vi "Proyecto 1 Control de Entrada.vi"() -> ()   [LabVIEW 2015]
panel:
  in  "Tab Control":T1(tab)
  in  "stop":bool
  out "Entradas/Salidas":i64
  out "Entrada":bool=TRUE
  out "Salida":bool=TRUE
  in  "Ajuste de Apertura":i32(knob)=3 scale=0.0..10.0
  in  "Control de Velocidad":i16(knob)=5 scale=0.0..10.0
  in  "Tiempo de espera":i16(knob)=1 scale=0.0..10.0
  # "Control Automatizado de Entrada"
  # "Componentes utilizados:\n      -Resistencias: 330 Ohms x2, 2.2 KOhms x2 a 1/2 watt\n      -Sensor infrarrojo y receptor infrarrojo\n      -LM293D(Puente H)\n      -Motor a pasos: M42SP-6TG (12 volts)\n      -Fuente de alimentación dual de 5 y 12 Volts"
  # "Serrano Bermúdez Luis Esteban"
  # "4/5/2019"
  # "Control de Entradas/Salidas a travez\nde sensores infrarrojos de obstrucción\ny de un motor a pasos que es controlado\na partir de un módulo LM293D (Conocido\ncomunmente como puente H)"
  # "Tiempo de Espera: Controla el tiempo que \npermanecerá abierta la puerta.\nControl de Velocidad: Ajusta la velocidad\ncon la que se mueve el motor a pasos.\nAjuste de Apertura: Modifica el grado de\napertura de la puerta permitiendo poder\naplicarlo a diferentes tipos de puertas"
  # "Entrada: Luz indicadora si se puede avanzar\na entrar o salir.\nSalida: Luz indicadora si se puede avanzar\na entrar o salir."
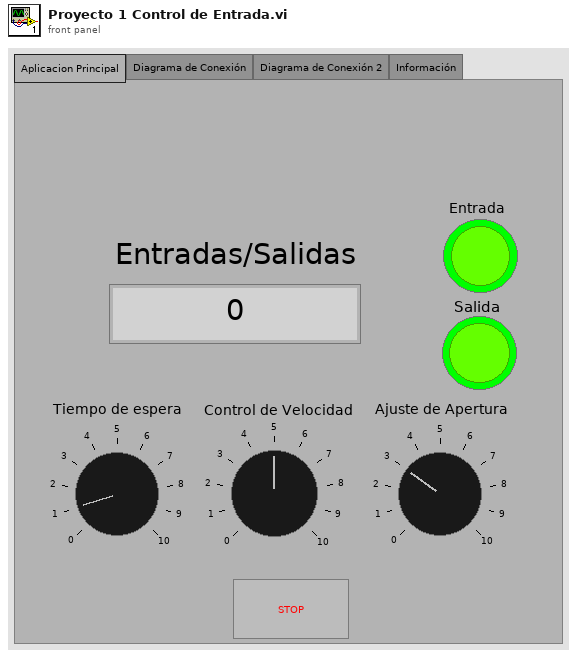
[diagram p1: front panel]
types:
  T1 = enum32{"Aplicacion Principal", "Diagrama de Conexión", "Diagrama de Conexión 2", "Información"}
  T2 = enum16{"Estado 0", "Estado 1", "Estado 2", "Estado 3"}
  T3 = enum16{"Estado 0", "Estado 1", "Estado 2", "Estado 3", "Estado 4", "Estado 5"}
  T4 = enum16{"Estado 0", "Estado 1", "Estado 2", "Estado 3", "Estado 4", "Estado 5", "Estado 6", "Estado 7", "Estado 8", "Estado 9"}
  T5 = enum16{"Estado 0", "Estado 1", "Estado 2", "Estado 3", "Estado 4", "Estado 5"}[]
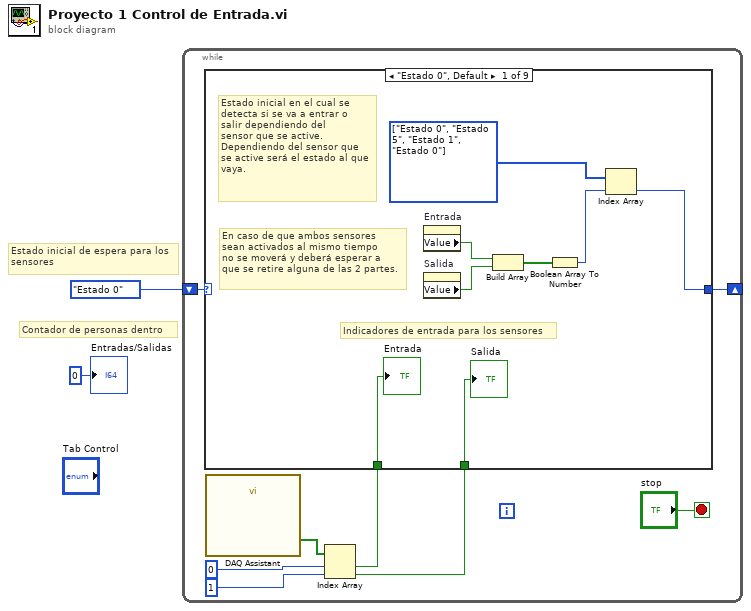
[diagram p0: block diagram]
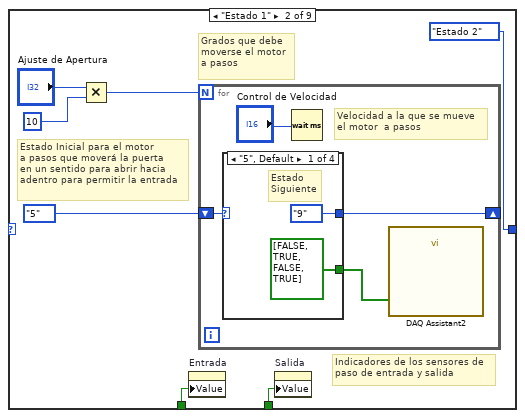
[diagram p2: hidden frame]
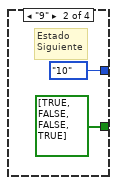
[diagram p3: hidden frame]
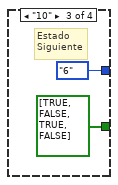
[diagram p4: hidden frame]
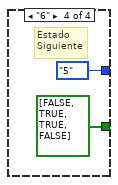
[diagram p5: hidden frame]
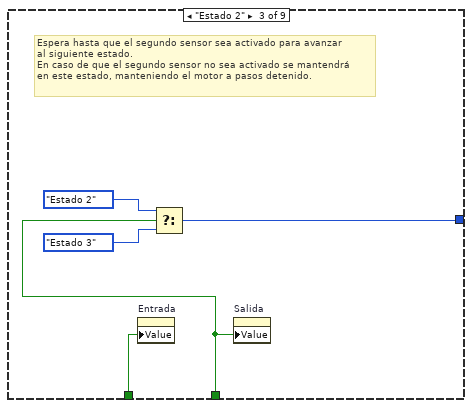
[diagram p6: hidden frame]
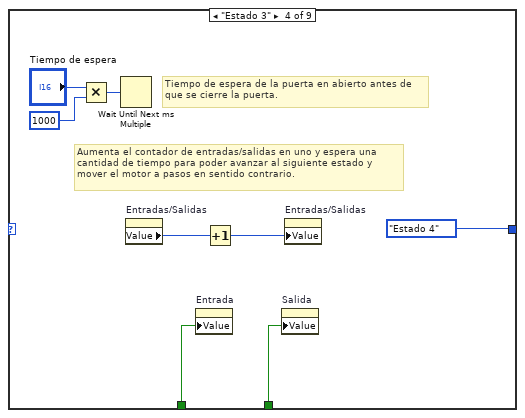
[diagram p7: hidden frame]
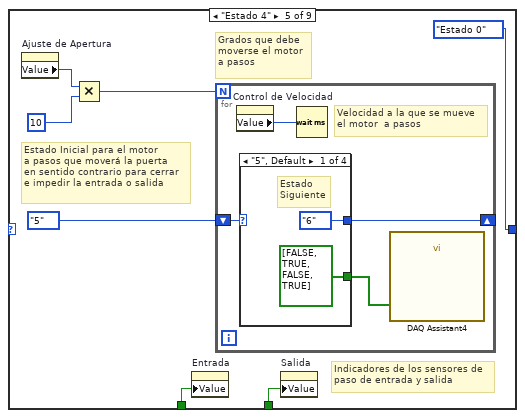
[diagram p8: hidden frame]
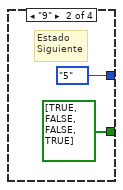
[diagram p9: hidden frame]
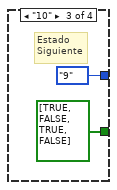
[diagram p10: hidden frame]
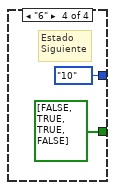
[diagram p11: hidden frame]
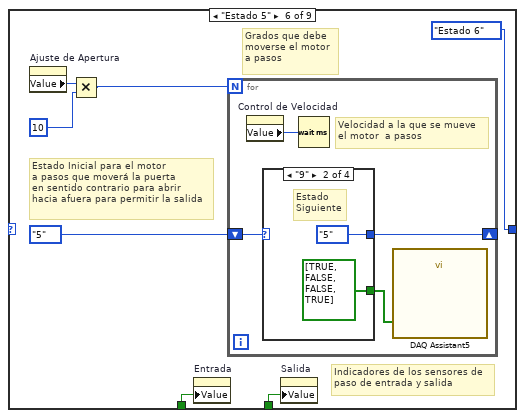
[diagram p12: hidden frame]
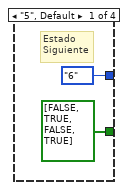
[diagram p13: hidden frame]
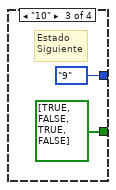
[diagram p14: hidden frame]
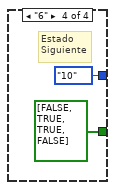
[diagram p15: hidden frame]
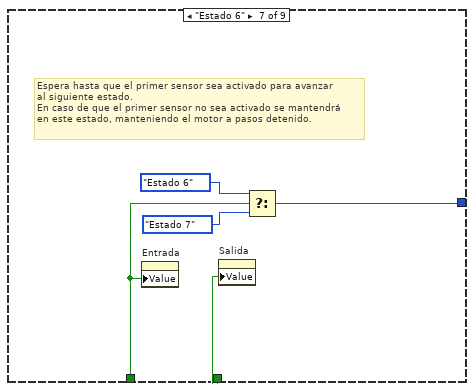
[diagram p16: hidden frame]
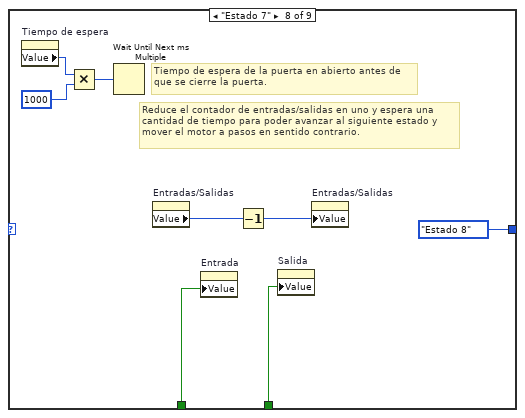
[diagram p17: hidden frame]
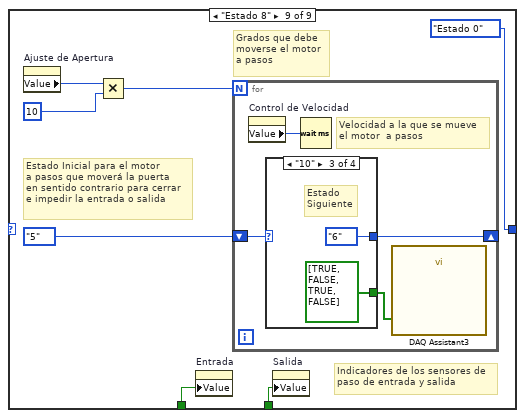
[diagram p18: hidden frame]
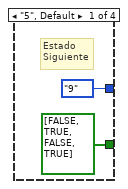
[diagram p19: hidden frame]
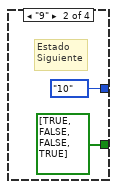
[diagram p20: hidden frame]
diagram:
  # "Contador de personas dentro"
  # "Estado inicial de espera para los\nsensores"
  n1 = while {
    shift-right: [w9] -> _
    shift-left: T2."Estado 0" -> [w10]
    stop <- "stop" stop-if-true
    n2 = call "DAQ Assistant"() -> ("data"=w5:bool[])  [unwired: 17 in, 2 out]
    n3 = Index Array(array=w5, index #1=0 ("index"), index #2=1 ("index")) -> (element #1=w4:bool, element #2=w3:bool)
    n4 = case shown="\"Estado 0\", Default" w10 {
      tunnel: [w18 T2."Estado 2" w40 T3."Estado 4" T4."Estado 0" T4."Estado 6" w91 T4."Estado 8" T4."Estado 0"] -> w9
      tunnel: w4 -> [w17 w19 w38 w46 w52 w70 w90 w97 w102]
      tunnel: w3 -> [w16 w20 w39 w47 w51 w71 w89 w98 w103]
      frame "Estado 0", Default {
        w15 = T5 [enum."Estado 0", enum."Estado 5", enum."Estado 1", enum."Estado 0"] items=["Estado 0", "Estado 1", "Estado 2", "Estado 3", "Estado 4", "Estado 5"]
        # "Indicadores de entrada para los sensores"
        # "En caso de que ambos sensores\nsean activados al mismo tiempo\nno se moverá y deberá esperar a\nque se retire alguna de las 2 partes."
        # "Estado inicial en el cual se\ndetecta si se va a entrar o\nsalir dependiendo del \nsensor que se active.\nDependiendo del sensor que\nse active será el estado al que\nvaya."
        n5 = property on="Entrada" class="Bool (strict)"() -> ("Value"=w12:bool)  [unwired: 2 in, 2 out]
        n6 = property on="Salida" class="Bool (strict)"() -> ("Value"=w11:bool)  [unwired: 2 in, 2 out]
        n7 = Build Array(w12, w11) -> (w13:bool[])
        n8 = Boolean Array To Number(Boolean array=w13) -> (number=w14:u32)
        n9 = Index Array(array=w15, index=w14) -> (element=w18:T3)
        "Entrada" <- w17
        "Salida" <- w16
      }
      frame "Estado 1" {
        # "Indicadores de los sensores de\npaso de entrada y salida"
        # "Grados que debe moverse el motor a pasos"
        # "Estado Inicial para el motor \na pasos que moverá la puerta\nen un sentido para abrir hacia\nadentro para permitir la entrada"
        n10 = Multiply(x="Ajuste de Apertura", y=10) -> (x*y=w23:i32)
        n11 = property on="Entrada" class="Bool (strict)"("Value"=w19) -> ()  [unwired: 2 in, 2 out]
        n12 = for {
          N: w23 -> [_]
          shift-right: [w28] -> _
          shift-left: enum16{"5", "9", "10", "6"}."5" -> [w29]
          # "Velocidad a la que se mueve\nel motor  a pasos"
          n13 = case shown="\"5\", Default" w29 {
            tunnel: [bool[] [FALSE, TRUE, FALSE, TRUE] bool[] [TRUE, FALSE, FALSE, TRUE] bool[] [TRUE, FALSE, TRUE, FALSE] bool[] [FALSE, TRUE, TRUE, FALSE]] -> w27
            tunnel: [enum16{"5", "9", "10", "6"}."9" enum16{"5", "9", "10", "6"}."10" enum16{"5", "9", "10", "6"}."6" enum16{"5", "9", "10", "6"}."5"] -> w28
            frame "5", Default {
              # "Estado\nSiguiente"
            }
            frame "9" {
              # "Estado\nSiguiente"
            }
            frame "10" {
              # "Estado\nSiguiente"
            }
            frame "6" {
              # "Estado\nSiguiente"
            }
          }
          n14 = Wait (ms)(milliseconds to wait="Control de Velocidad") -> ()  [unwired: 1 out]
          n15 = call "DAQ Assistant2"("data"=w27) -> ()  [unwired: 17 in, 2 out]
        }
        n16 = property on="Salida" class="Bool (strict)"("Value"=w20) -> ()  [unwired: 2 in, 2 out]
      }
      frame "Estado 2" {
        # "Espera hasta que el segundo sensor sea activado para avanzar\nal siguiente estado.\nEn caso de que el segundo sensor no sea activado se mantendrá\nen este estado, manteniendo el motor a pasos detenido."
        n17 = property on="Entrada" class="Bool (strict)"("Value"=w38) -> ()  [unwired: 2 in, 2 out]
        n18 = Select(t=T2."Estado 2", s=w39, f=T2."Estado 3") -> (s? t:f=w40:T2)
        n19 = property on="Salida" class="Bool (strict)"("Value"=w39) -> ()  [unwired: 2 in, 2 out]
      }
      frame "Estado 3" {
        # "Tiempo de espera de la puerta en abierto antes de\nque se cierre la puerta."
        # "Aumenta el contador de entradas/salidas en uno y espera una\ncantidad de tiempo para poder avanzar al siguiente estado y\nmover el motor a pasos en sentido contrario."
        n20 = Multiply(x="Tiempo de espera", y=1000) -> (x*y=w43:i32)
        n21 = Wait Until Next ms Multiple(millisecond multiple=w43) -> ()  [unwired: 1 out]
        n22 = property on="Entradas/Salidas" class="DigNum (strict)"() -> ("Value"=w48:i64)  [unwired: 2 in, 2 out]
        n23 = property on="Entrada" class="Bool (strict)"("Value"=w46) -> ()  [unwired: 2 in, 2 out]
        n24 = Increment(x=w48) -> (x+1=w49:i64)
        n25 = property on="Salida" class="Bool (strict)"("Value"=w47) -> ()  [unwired: 2 in, 2 out]
        n26 = property on="Entradas/Salidas" class="DigNum (strict)"("Value"=w49) -> ()  [unwired: 2 in, 2 out]
      }
      frame "Estado 4" {
        # "Indicadores de los sensores de\npaso de entrada y salida"
        # "Estado Inicial para el motor \na pasos que moverá la puerta\nen sentido contrario para cerrar\ne impedir la entrada o salida"
        # "Grados que debe moverse el motor a pasos"
        n27 = property on="Ajuste de Apertura" class="Knob (strict)"() -> ("Value"=w53:i32)  [unwired: 2 in, 2 out]
        n28 = Multiply(x=w53, y=10) -> (x*y=w55:i32)
        n29 = property on="Entrada" class="Bool (strict)"("Value"=w52) -> ()  [unwired: 2 in, 2 out]
        n30 = for {
          N: w55 -> [_]
          shift-right: [w60] -> _
          shift-left: enum16{"5", "9", "10", "6"}."5" -> [w61]
          # "Velocidad a la que se mueve\nel motor  a pasos"
          n31 = property on="Control de Velocidad" class="Knob (strict)"() -> ("Value"=w58:i16)  [unwired: 2 in, 2 out]
          n32 = case shown="\"5\", Default" w61 {
            tunnel: [bool[] [FALSE, TRUE, FALSE, TRUE] bool[] [TRUE, FALSE, FALSE, TRUE] bool[] [TRUE, FALSE, TRUE, FALSE] bool[] [FALSE, TRUE, TRUE, FALSE]] -> w59
            tunnel: [enum16{"5", "9", "10", "6"}."6" enum16{"5", "9", "10", "6"}."5" enum16{"5", "9", "10", "6"}."9" enum16{"5", "9", "10", "6"}."10"] -> w60
            frame "5", Default {
              # "Estado\nSiguiente"
            }
            frame "9" {
              # "Estado\nSiguiente"
            }
            frame "10" {
              # "Estado\nSiguiente"
            }
            frame "6" {
              # "Estado\nSiguiente"
            }
          }
          n33 = Wait (ms)(milliseconds to wait=w58) -> ()  [unwired: 1 out]
          n34 = call "DAQ Assistant4"("data"=w59) -> ()  [unwired: 17 in, 2 out]
        }
        n35 = property on="Salida" class="Bool (strict)"("Value"=w51) -> ()  [unwired: 2 in, 2 out]
      }
      frame "Estado 5" {
        # "Indicadores de los sensores de\npaso de entrada y salida"
        # "Estado Inicial para el motor \na pasos que moverá la puerta\nen sentido contrario para abrir\nhacia afuera para permitir la salida"
        # "Grados que debe moverse el motor a pasos"
        n36 = property on="Ajuste de Apertura" class="Knob (strict)"() -> ("Value"=w72:i32)  [unwired: 2 in, 2 out]
        n37 = Multiply(x=w72, y=10) -> (x*y=w74:i32)
        n38 = property on="Entrada" class="Bool (strict)"("Value"=w70) -> ()  [unwired: 2 in, 2 out]
        n39 = for {
          N: w74 -> [_]
          shift-right: [w79] -> _
          shift-left: enum16{"5", "9", "10", "6"}."5" -> [w80]
          # "Velocidad a la que se mueve\nel motor  a pasos"
          n40 = property on="Control de Velocidad" class="Knob (strict)"() -> ("Value"=w77:i16)  [unwired: 2 in, 2 out]
          n41 = case shown="\"9\"" w80 {
            tunnel: [bool[] [FALSE, TRUE, FALSE, TRUE] bool[] [TRUE, FALSE, FALSE, TRUE] bool[] [TRUE, FALSE, TRUE, FALSE] bool[] [FALSE, TRUE, TRUE, FALSE]] -> w78
            tunnel: [enum16{"5", "9", "10", "6"}."6" enum16{"5", "9", "10", "6"}."5" enum16{"5", "9", "10", "6"}."9" enum16{"5", "9", "10", "6"}."10"] -> w79
            frame "5", Default {
              # "Estado\nSiguiente"
            }
            frame "9" {
              # "Estado\nSiguiente"
            }
            frame "10" {
              # "Estado\nSiguiente"
            }
            frame "6" {
              # "Estado\nSiguiente"
            }
          }
          n42 = Wait (ms)(milliseconds to wait=w77) -> ()  [unwired: 1 out]
          n43 = call "DAQ Assistant5"("data"=w78) -> ()  [unwired: 17 in, 2 out]
        }
        n44 = property on="Salida" class="Bool (strict)"("Value"=w71) -> ()  [unwired: 2 in, 2 out]
      }
      frame "Estado 6" {
        # "Espera hasta que el primer sensor sea activado para avanzar\nal siguiente estado.\nEn caso de que el primer sensor no sea activado se mantendrá\nen este estado, manteniendo el motor a pasos detenido."
        n45 = property on="Entrada" class="Bool (strict)"("Value"=w90) -> ()  [unwired: 2 in, 2 out]
        n46 = property on="Salida" class="Bool (strict)"("Value"=w89) -> ()  [unwired: 2 in, 2 out]
        n47 = Select(t=T4."Estado 6", s=w90, f=T4."Estado 7") -> (s? t:f=w91:T4)
      }
      frame "Estado 7" {
        # "Tiempo de espera de la puerta en abierto antes de\nque se cierre la puerta."
        # "Reduce el contador de entradas/salidas en uno y espera una\ncantidad de tiempo para poder avanzar al siguiente estado y\nmover el motor a pasos en sentido contrario."
        n48 = property on="Tiempo de espera" class="Knob (strict)"() -> ("Value"=w95:i16)  [unwired: 2 in, 2 out]
        n49 = Multiply(x=w95, y=1000) -> (x*y=w94:i32)
        n50 = Wait Until Next ms Multiple(millisecond multiple=w94) -> ()  [unwired: 1 out]
        n51 = property on="Entradas/Salidas" class="DigNum (strict)"() -> ("Value"=w100:i64)  [unwired: 2 in, 2 out]
        n52 = property on="Entrada" class="Bool (strict)"("Value"=w97) -> ()  [unwired: 2 in, 2 out]
        n53 = Decrement(x=w100) -> (x-1=w101:i64)
        n54 = property on="Salida" class="Bool (strict)"("Value"=w98) -> ()  [unwired: 2 in, 2 out]
        n55 = property on="Entradas/Salidas" class="DigNum (strict)"("Value"=w101) -> ()  [unwired: 2 in, 2 out]
      }
      frame "Estado 8" {
        # "Estado Inicial para el motor \na pasos que moverá la puerta\nen sentido contrario para cerrar\ne impedir la entrada o salida"
        # "Indicadores de los sensores de\npaso de entrada y salida"
        # "Grados que debe moverse el motor a pasos"
        n56 = property on="Ajuste de Apertura" class="Knob (strict)"() -> ("Value"=w104:i32)  [unwired: 2 in, 2 out]
        n57 = Multiply(x=w104, y=10) -> (x*y=w106:i32)
        n58 = property on="Entrada" class="Bool (strict)"("Value"=w102) -> ()  [unwired: 2 in, 2 out]
        n59 = for {
          N: w106 -> [_]
          shift-right: [w111] -> _
          shift-left: enum16{"5", "9", "10", "6"}."5" -> [w112]
          # "Velocidad a la que se mueve\nel motor  a pasos"
          n60 = property on="Control de Velocidad" class="Knob (strict)"() -> ("Value"=w109:i16)  [unwired: 2 in, 2 out]
          n61 = case shown="\"10\"" w112 {
            tunnel: [bool[] [FALSE, TRUE, FALSE, TRUE] bool[] [TRUE, FALSE, FALSE, TRUE] bool[] [TRUE, FALSE, TRUE, FALSE] bool[] [FALSE, TRUE, TRUE, FALSE]] -> w110
            tunnel: [enum16{"5", "9", "10", "6"}."9" enum16{"5", "9", "10", "6"}."10" enum16{"5", "9", "10", "6"}."6" enum16{"5", "9", "10", "6"}."5"] -> w111
            frame "5", Default {
              # "Estado\nSiguiente"
            }
            frame "9" {
              # "Estado\nSiguiente"
            }
            frame "10" {
              # "Estado\nSiguiente"
            }
            frame "6" {
              # "Estado\nSiguiente"
            }
          }
          n62 = Wait (ms)(milliseconds to wait=w109) -> ()  [unwired: 1 out]
          n63 = call "DAQ Assistant3"("data"=w110) -> ()  [unwired: 17 in, 2 out]
        }
        n64 = property on="Salida" class="Bool (strict)"("Value"=w103) -> ()  [unwired: 2 in, 2 out]
      }
    }
  }
  "Entradas/Salidas" <- i64 0 ("Entradas/Salidas")
